vi "main_PG.vi"() -> ()   [LabVIEW 2017]
panel:
  out "P2":dbl[](array[numeric])
  out "T2":dbl[](array[numeric])
  out "V":dbl[](array[numeric])
  out "P1":dbl[](array[numeric])
  in  "Heater 2":bool
  in  "Tab Control 2":enum32{"Page 1", "Page 2"}(tab)
  in  "ON/OFF Control Loop":bool caption="Start"
  in  "Ring":u16(ring) items=["Isothermal Process", "Isochoric Process", "Boyle's Law", "Gay-Lussac Law", ""]
  in  "Exit":bool
  out "NI1":tag caption="NI device"
  out "Compressor":bool
  out "Heater":bool
  in  "Tab Control":enum32{"Page 1", "Page 2", "Page 3", "Page 4"}(tab)
  out "Air Volume (L)":dbl format="%#_3f"
  out "process":string
  in  "Save as image 6":bool
  in  "Save as Excel 6":bool
  in  "Pause Button 6":bool
  in  "Reset Chart 6":bool
  out "PV Graph":cluster{dbl[], dbl[]}(graph)
  out "Waveform Chart":cluster{"Scalar":dbl, "Scalar":dbl}(graph)
  out "Temperature":dbl(slide) caption="Temperature [C]" scale=0.0..100.0
  out "Pressure":dbl(knob) caption="Pressure [bar]" scale=-1.0..6.0
  out "Tank1":dbl(slide) scale=0.0..4.0
  in  "Save as image 5":bool
  in  "Save as Excel 5":bool
  in  "Pause Button 5":bool
  in  "Reset Chart 5":bool
  in  "Reset Chart 4":bool
  in  "Pause Button 4":bool
  in  "Save as Excel 4":bool
  in  "Save as image 4":bool
  out "Tank1 2":dbl(slide) scale=0.0..4.0
  out "Pressure 2":dbl(knob) caption="Pressure [bar]" scale=-1.0..6.0 scale format="%#_3f"
  out "Temperature 2":dbl(slide) caption="Temperature [C]" scale=0.0..100.0
  out "Waveform Chart 2":cluster{"Scalar":dbl, "Scalar":dbl}(graph)
  out "PT Graph":cluster{dbl[], dbl[]}(graph)
  in  "Reset Chart 3":bool
  in  "Pause Button 3":bool
  in  "Save as Excel 3":bool
  in  "Save as image 3":bool
  out "String":string
  out "Table":string[][](table)
  in  "BoyleNum":i64 caption="Number of samples"
  out "Total Samples":i32
  in  "BoyleNum 2":i64 caption="Number of samples"
  out "Total Samples 2":i32 caption="Total Samples"
  out "Table 2":string[][](table)
  out "String 2":string
  in  "Tab Control 3":enum32{"Page 1", "Page 2"}(tab)
  # "Expansion Processes of a Perfect Gas"
  # "Liquid Volume (L)"
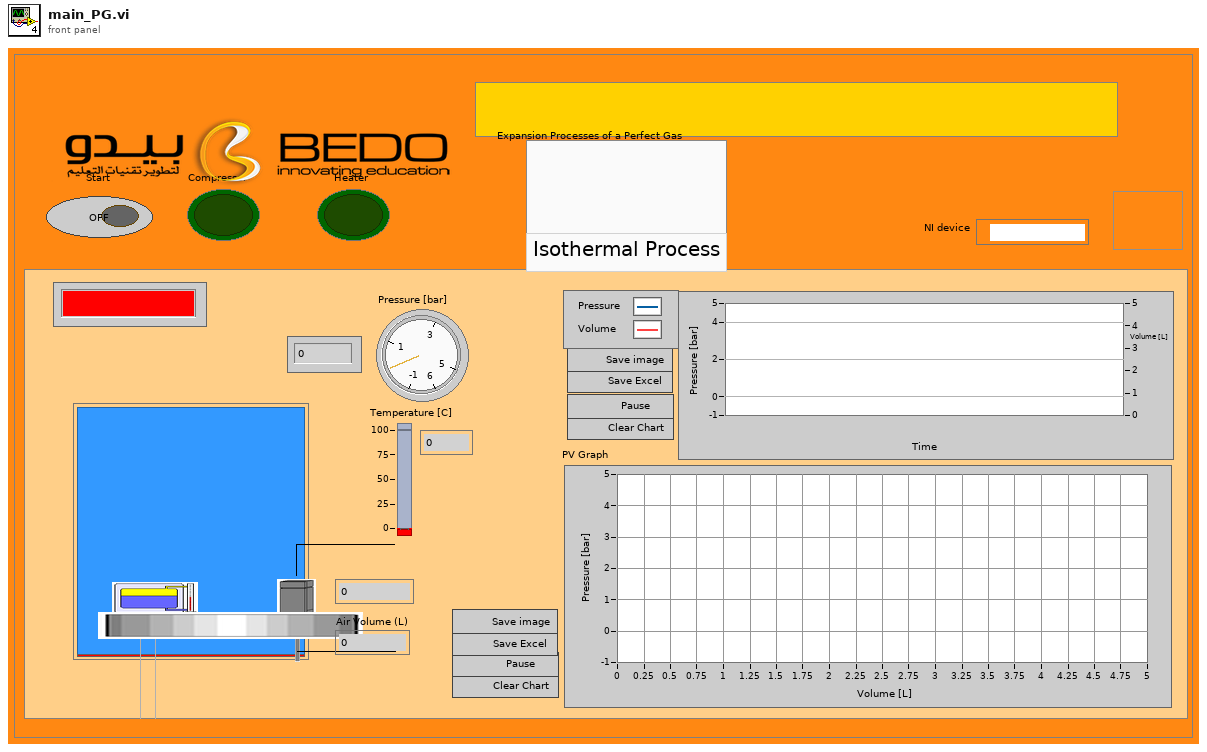
[diagram p1: front panel]
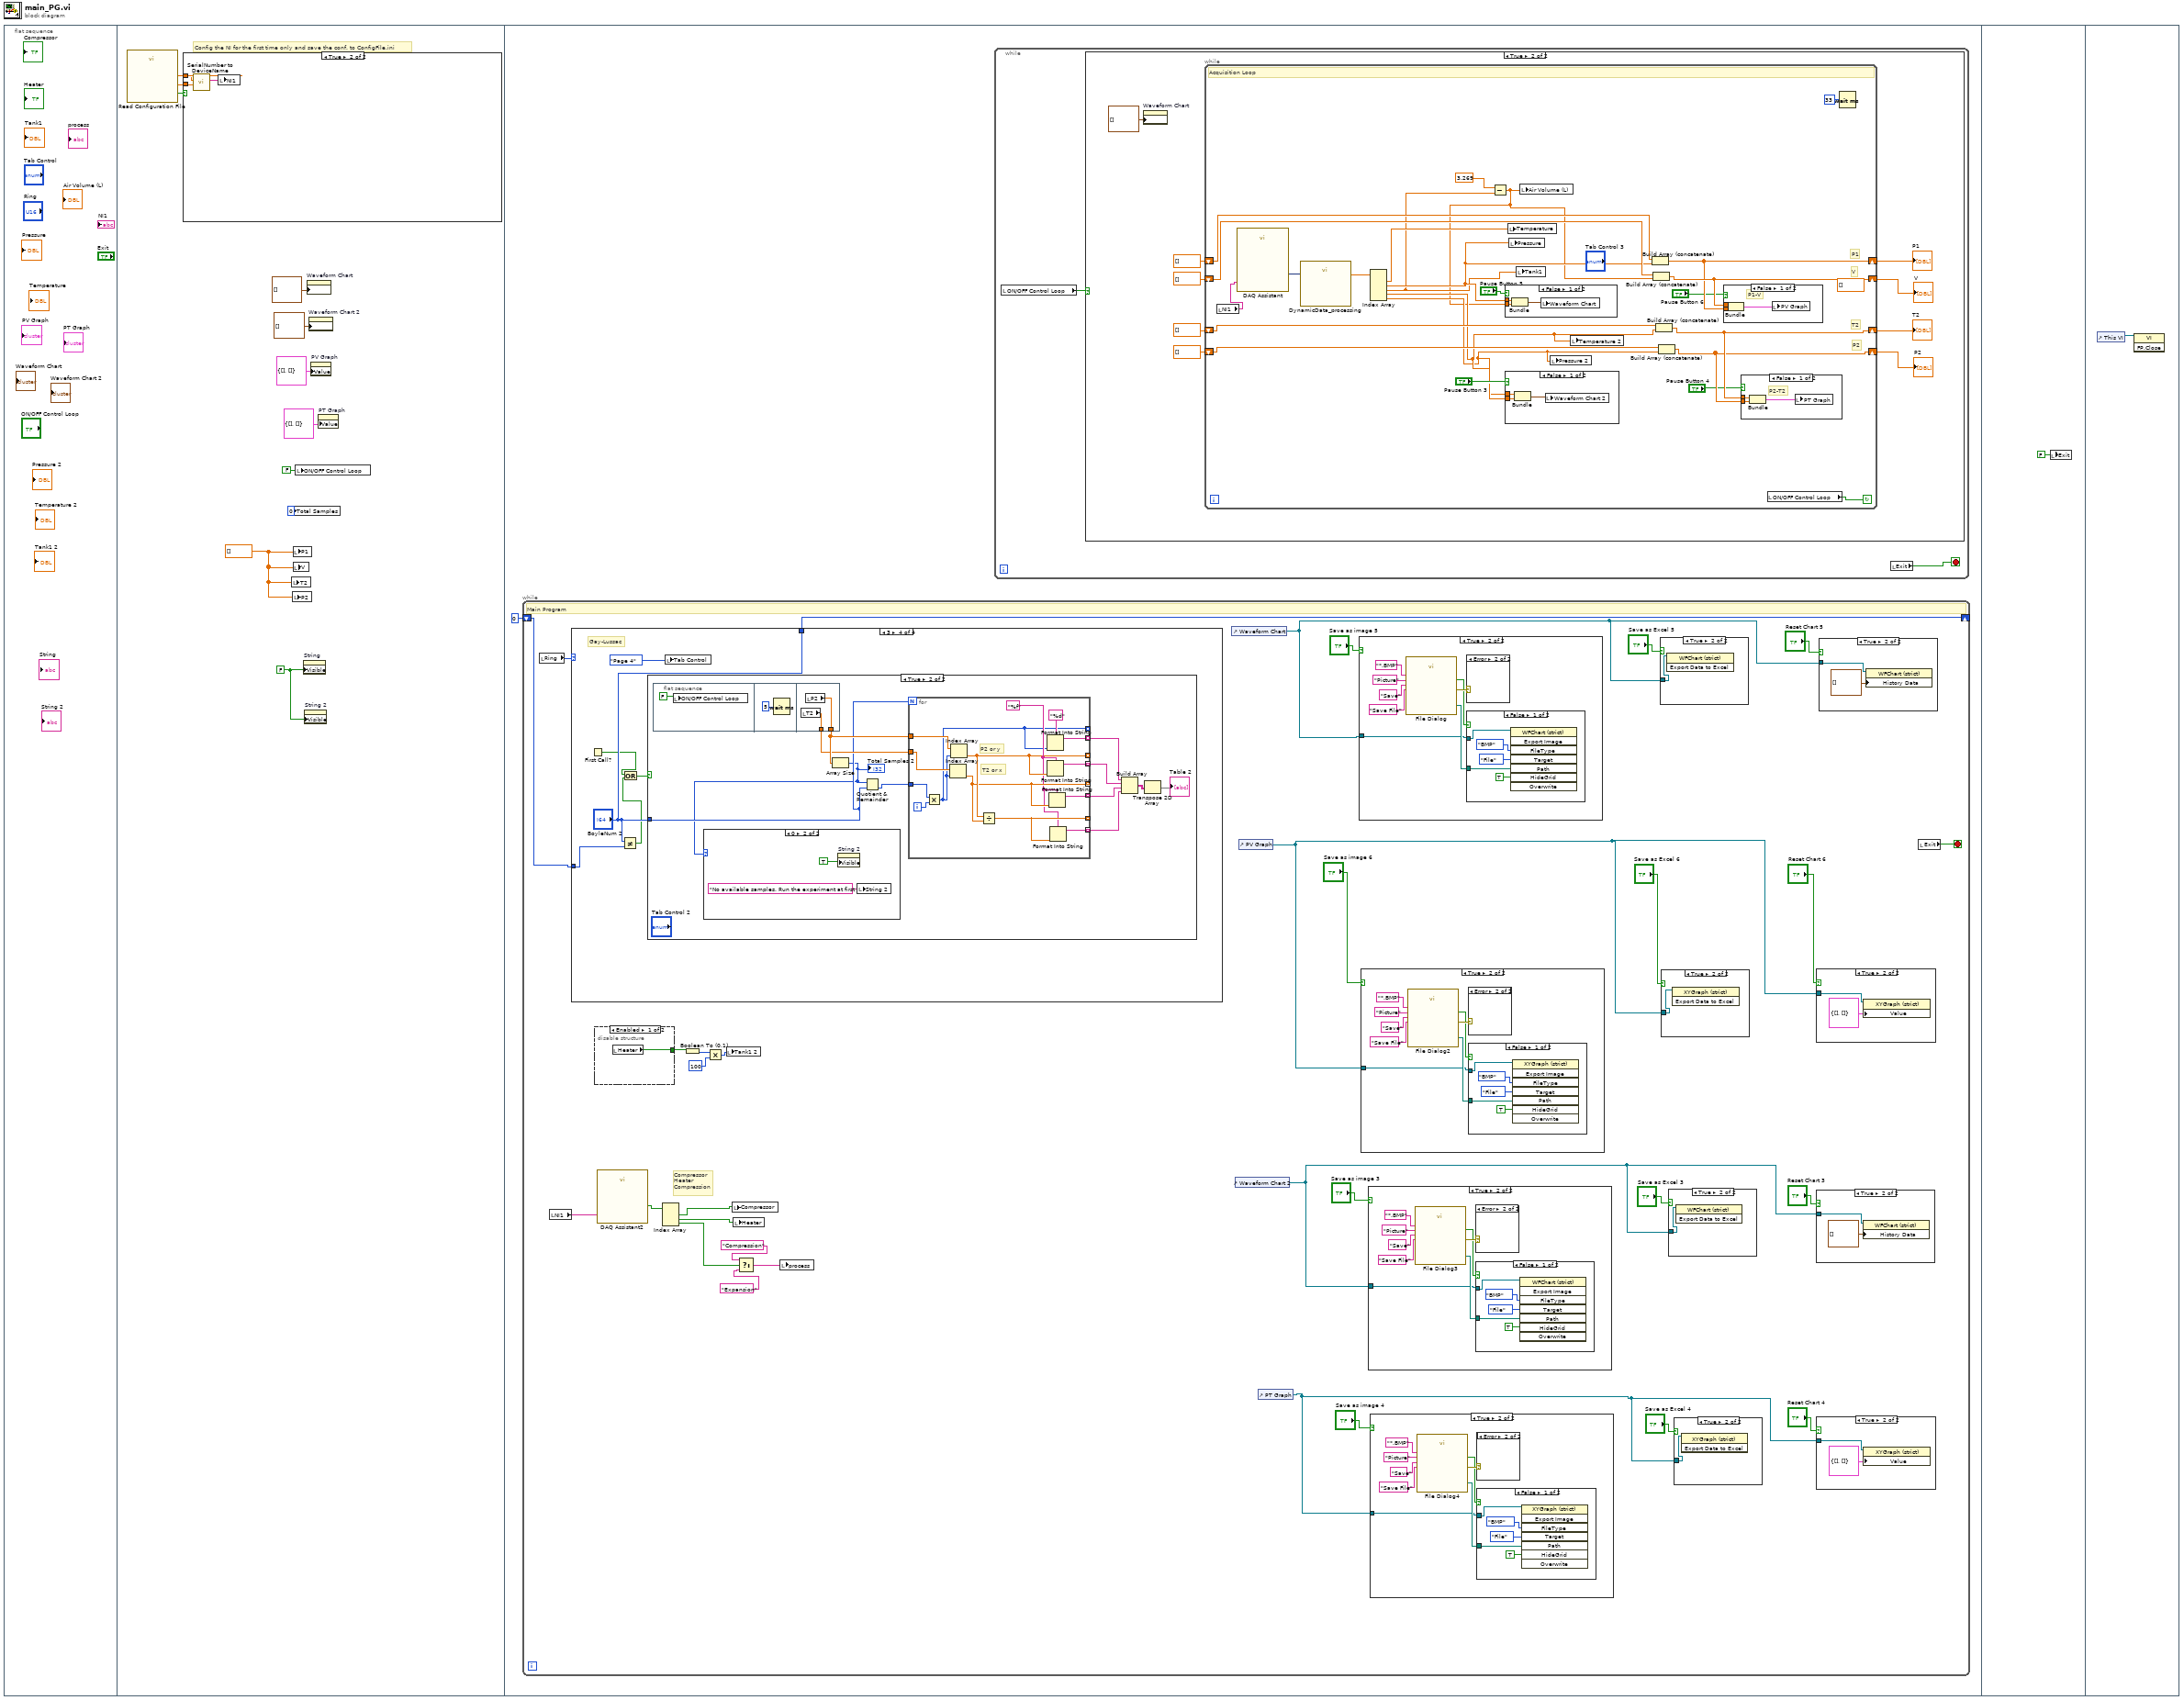
[diagram p0: block diagram]
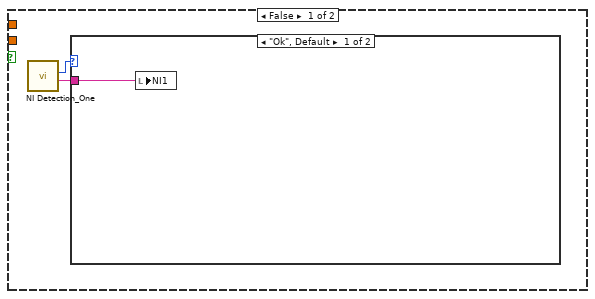
[diagram p2: hidden frame]
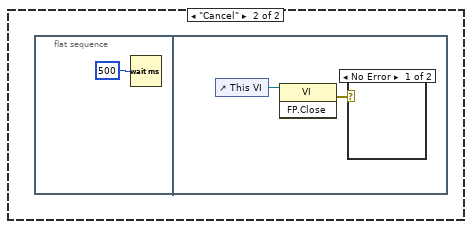
[diagram p3: hidden frame]
diagram:
  n1 = flat-sequence {
    frame #0 {
    }
    frame #1 {
      w1 = FALSE ("Visible")
      w2 = dbl[] [] ("Array")
      # "Config the NI for the first time only and save the conf. to ConfigFile.ini"
      n2 = call "Read Configuration File.vi"() -> ("Serial Numbers Found"=w9:bool, "NI1"=w10:dbl, "NI2"=w11:dbl)  [unwired: 13 in]
      n3 = case shown="True" w9 {
        tunnel: w10 -> [_ w20]
        tunnel: w11 -> [_ w19]
        frame False {
          n4 = call "NI Detection_One.vi"() -> ("NI 1"=w12:tag, "Ok/Cancel"=w13:enum16{"Ok", "Cancel"})  [unwired: 8 in, 1 out]
          n5 = case shown="\"Ok\", Default" w13 {
            tunnel: w12 -> [w14 _]
            frame "Ok", Default {
              n6 = local write "NI1"(w14) -> ()
            }
            frame "Cancel" {
              n7 = flat-sequence {
                frame #0 {
                  n8 = Wait (ms)(milliseconds to wait=u32 500) -> ()  [unwired: 1 out]
                }
                frame #1 {
                  n9 = control-ref of="This VI"() -> (w17:refnum<vi>)
                  n10 = invoke class="VI" method="FP.Close"(reference=w17) -> (error out=w16:errorcluster)  [unwired: 2 in, 2 out]
                  n11 = case shown="No Error" w16 {
                    frame No Error {
                    }
                    frame Error {
                    }
                  }
                }
              }
            }
          }
        }
        frame True {
          n12 = call "SerialNumber to DeviceName.vi"("NI2 Serial Number"=w19, "NI1 Serial Number"=w20) -> ("NI1 Device Name"=w18:tag)  [unwired: 8 in, 1 out]
          n13 = local write "NI1"(w18) -> ()
        }
      }
      n14 = local write "Total Samples"(0 ("size(s)")) -> ()
      n15 = local write "T2"(w2) -> ()
      n16 = local write "P2"(w2) -> ()
      n17 = local write "P1"(w2) -> ()
      n18 = local write "V"(w2) -> ()
      n19 = local write "ON/OFF Control Loop"(FALSE ("ON/OFF Control Loop")) -> ()
      n20 = property on="String" class="Str"("Visible"=w1) -> ()  [unwired: 2 in, 2 out]
      n21 = property on="String 2" class="Str"("Visible"=w1) -> ()  [unwired: 2 in, 2 out]
      n22 = property on="Waveform Chart" class="WFChart (strict)"("History Data"=cluster{"Scalar":dbl, "Scalar":dbl}[] []) -> ()  [unwired: 2 in, 2 out]
      n23 = property on="Waveform Chart 2" class="WFChart (strict)"("History Data"=cluster{"Scalar":dbl, "Scalar":dbl}[] []) -> ()  [unwired: 2 in, 2 out]
      n24 = property on="PV Graph" class="XYGraph (strict)"("Value"=cluster{dbl[], dbl[]} {[], []} ("PV Graph")) -> ()  [unwired: 2 in, 2 out]
      n25 = property on="PT Graph" class="XYGraph (strict)"("Value"=cluster{dbl[], dbl[]} {[], []} ("PT Graph")) -> ()  [unwired: 2 in, 2 out]
    }
    frame #2 {
      n26 = while {
        shift-right: [w31] -> _
        shift-left: i64 0 ("BoyleNum") -> [w30]
        stop <- w53 stop-if-true
        # "Compressor\nHeater\nCompression"
        # "Main Program"
        n27 = local read "Ring"() -> (w52:u16)
        n28 = local read "NI1"() -> (w29:tag)
        n29 = case shown="3" w52 {
          tunnel: [w120 w122 "BoyleNum" "BoyleNum 2"] -> w31
          tunnel: w30 -> [w120 w122 w127 w165]
          frame 0, Default {
            n30 = local write "Tab Control"(enum32{"Page 1", "Page 2"}."Page 1" ("Tab Control")) -> ()
          }
          frame 1 {
            n31 = local write "Tab Control"(enum32{"Page 1", "Page 2"}."Page 2" ("Tab Control")) -> ()
          }
          frame 2 {
            # "Boyle"
            n32 = First Call?() -> (First Call?: T/F=w124:bool)
            n33 = Not Equal?(x="BoyleNum", y=w127) -> (x != y?=w126:bool)
            n34 = Or(x=w124, y=w126) -> (x .or. y?=w125:bool)
            n35 = case shown="True" w125 {
              tunnel: "BoyleNum" -> [_ w132]
              frame False {
              }
              frame True {
                n36 = flat-sequence {
                  tunnel: [w161] -> w139
                  tunnel: [w160] -> w138
                  frame #0 {
                    n37 = local write "ON/OFF Control Loop"(FALSE ("ON/OFF Control Loop")) -> ()
                  }
                  frame #1 {
                    n38 = Wait (ms)(milliseconds to wait=u32 5) -> ()  [unwired: 1 out]
                  }
                  frame #2 {
                    n39 = local read "V"() -> (w160:dbl[])
                    n40 = local read "P1"() -> (w161:dbl[])
                  }
                }
                n41 = Array Size(array=w139) -> (size(s)=w130:i32)
                "Total Samples" <- w130
                n42 = case shown="0" w130 {
                  frame 1, Default {
                    n43 = property on="String" class="Str"("Visible"=FALSE) -> ()  [unwired: 2 in, 2 out]
                  }
                  frame 0 {
                    n44 = property on="String" class="Str"("Visible"=TRUE) -> ()  [unwired: 2 in, 2 out]
                    n45 = local write "String"("No available samples. Run the experiment at first !" ("String 2")) -> ()
                  }
                }
                n46 = Quotient & Remainder(x=w130, y=w132) -> (floor(x/y)=w140:i64)  [unwired: 1 out]
                n47 = for {
                  N: w132 -> [_]
                  tunnel: w140 -> [w157]
                  tunnel: w139 -> [w155]
                  tunnel: w138 -> [w154]
                  tunnel: [w152] -> _ mode=indexing
                  tunnel: [w150] -> _ mode=indexing
                  tunnel: [w146] -> _ mode=indexing
                  tunnel: [w149] -> _ mode=indexing
                  tunnel: [w148] -> w137 mode=indexing
                  tunnel: [w153] -> w136 mode=indexing
                  tunnel: [w151] -> w135 mode=indexing
                  tunnel: [w145] -> w131 mode=indexing
                  i -> [w146]
                  w147 = "%f" ("format string")
                  # "V or x"
                  # "P1 or y"
                  n48 = Multiply(x=w157, y=w146) -> (x*y=w156:i64)
                  n49 = Index Array(array=w154, index=w156) -> (element=w150:dbl)
                  n50 = Index Array(array=w155, index=w156) -> (element=w152:dbl)
                  n51 = Multiply(x=w152, y=w150) -> (x*y=w149:dbl)
                  n52 = Format Into String(format string=w147, w152) -> (resulting string=w148:string)  [unwired: 2 in, 1 out]
                  n53 = Format Into String(format string="%d", w146) -> (resulting string=w145:string)  [unwired: 2 in, 1 out]
                  n54 = Format Into String(format string=w147, w150) -> (resulting string=w153:string)  [unwired: 2 in, 1 out]
                  n55 = Format Into String(format string=w147, w149) -> (resulting string=w151:string)  [unwired: 2 in, 1 out]
                }
                n56 = Build Array(w131, w137, w136, w135) -> (w134:string[][])
                n57 = Transpose 2D Array(2D array=w134) -> (transposed array=→"Table":string[][])
              }
            }
            n58 = local write "Tab Control"(enum32{"Page 1", "Page 2", "Page 3", "Page 4"}."Page 3" ("Tab Control")) -> ()
          }
          frame 3 {
            # "Gay-Lussac"
            n59 = First Call?() -> (First Call?: T/F=w162:bool)
            n60 = Not Equal?(x="BoyleNum 2", y=w165) -> (x != y?=w164:bool)
            n61 = Or(x=w162, y=w164) -> (x .or. y?=w163:bool)
            n62 = case shown="True" w163 {
              tunnel: "BoyleNum 2" -> [_ w170]
              frame False {
              }
              frame True {
                n63 = flat-sequence {
                  tunnel: [w199] -> w177
                  tunnel: [w198] -> w176
                  frame #0 {
                    n64 = local write "ON/OFF Control Loop"(FALSE ("ON/OFF Control Loop")) -> ()
                  }
                  frame #1 {
                    n65 = Wait (ms)(milliseconds to wait=u32 5) -> ()  [unwired: 1 out]
                  }
                  frame #2 {
                    n66 = local read "T2"() -> (w198:dbl[])
                    n67 = local read "P2"() -> (w199:dbl[])
                  }
                }
                n68 = Array Size(array=w177) -> (size(s)=w168:i32)
                "Total Samples 2" <- w168
                n69 = case shown="0" w168 {
                  frame 1, Default {
                    n70 = property on="String 2" class="Str"("Visible"=FALSE) -> ()  [unwired: 2 in, 2 out]
                  }
                  frame 0 {
                    n71 = property on="String 2" class="Str"("Visible"=TRUE) -> ()  [unwired: 2 in, 2 out]
                    n72 = local write "String 2"("No available samples. Run the experiment at first !" ("String 2")) -> ()
                  }
                }
                n73 = Quotient & Remainder(x=w168, y=w170) -> (floor(x/y)=w178:i64)  [unwired: 1 out]
                n74 = for {
                  N: w170 -> [_]
                  tunnel: w178 -> [w195]
                  tunnel: w177 -> [w194]
                  tunnel: w176 -> [w193]
                  tunnel: [w191] -> _ mode=indexing
                  tunnel: [w189] -> _ mode=indexing
                  tunnel: [w182] -> _ mode=indexing
                  tunnel: [w188] -> _ mode=indexing
                  tunnel: [w187] -> w175 mode=indexing
                  tunnel: [w192] -> w174 mode=indexing
                  tunnel: [w190] -> w173 mode=indexing
                  tunnel: [w184] -> w169 mode=indexing
                  i -> [w185]
                  w186 = "%f" ("format string")
                  # "T2 or x"
                  # "P2 or y"
                  n75 = Multiply(x=w195, y=w185) -> (x*y=w182:i64)
                  n76 = Index Array(array=w193, index=w182) -> (element=w189:dbl)
                  n77 = Index Array(array=w194, index=w182) -> (element=w191:dbl)
                  n78 = Divide(x=w191, y=w189) -> (x/y=w188:dbl)
                  n79 = Format Into String(format string=w186, w191) -> (resulting string=w187:string)  [unwired: 2 in, 1 out]
                  n80 = Format Into String(format string="%d", w182) -> (resulting string=w184:string)  [unwired: 2 in, 1 out]
                  n81 = Format Into String(format string=w186, w189) -> (resulting string=w192:string)  [unwired: 2 in, 1 out]
                  n82 = Format Into String(format string=w186, w188) -> (resulting string=w190:string)  [unwired: 2 in, 1 out]
                }
                n83 = Build Array(w169, w175, w174, w173) -> (w172:string[][])
                n84 = Transpose 2D Array(2D array=w172) -> (transposed array=→"Table 2":string[][])
              }
            }
            n85 = local write "Tab Control"(enum32{"Page 1", "Page 2", "Page 3", "Page 4"}."Page 4" ("Tab Control")) -> ()
          }
        }
        n86 = disable-structure shown="Enabled" {
          disable-tunnel: [w118 "Heater 2"] -> w51
          frame Enabled {
            n87 = local read "Heater"() -> (w118:bool)
          }
          frame Disabled {
          }
        }
        n88 = call "DAQ Assistant2"("device name"=w29) -> ("data"=w28:bool[])  [unwired: 16 in, 2 out]
        n89 = Index Array(array=w28) -> (element #1=w27:bool, element #2=w26:bool, element #3=w25:bool)  [unwired: 3 in]
        n90 = Boolean To (0,1)(Boolean=w51) -> (0, 1=w50:i16)
        n91 = Multiply(x=w50, y=i16 100) -> (x*y=w49:i16)
        n92 = local write "Tank1 2"(w49) -> ()
        n93 = local write "Compressor"(w27) -> ()
        n94 = local write "Heater"(w26) -> ()
        n95 = Select(t="Compression", s=w25, f="Expansion") -> (s? t:f=w22:string)
        n96 = local write "process"(w22) -> ()
        n97 = control-ref of="Waveform Chart"() -> (w46:refnum<vi>)
        n98 = control-ref of="Waveform Chart 2"() -> (w36:refnum<vi>)
        n99 = control-ref of="PV Graph"() -> (w42:refnum<vi>)
        n100 = control-ref of="PT Graph"() -> (w32:refnum<vi>)
        n101 = case shown="True" "Save as image 5" {
          tunnel: w46 -> [_ w105]
          frame False {
          }
          frame True {
            n102 = call "File Dialog"("prompt"="Save File", "button label"="Save", "pattern (all files)"="*.BMP", "pattern label"="Picture") -> ("selected path"=w107:path, "cancelled"=w106:bool, "error out"=w108:errorcluster)  [unwired: 8 in, 1 out]
            n103 = case shown="Error" w108 {
              frame No Error {
              }
              frame Error {
              }
            }
            n104 = case shown="False" w106 {
              tunnel: w107 -> [w115 _]
              tunnel: w105 -> [w113 _]
              frame False {
                n105 = invoke on="Invoke Node" class="WFChart (strict)" method="Export Image"(reference=w113, "FileType"=enum32{"BMP", "EPS", "EMF", "PICT"}."BMP" ("File Type"), "Target"=enum32{"File", "Clipboard"}."File", "Path"=w115, "HideGrid"=TRUE ("Hide Grid")) -> ()  [unwired: 3 in, 8 out]
              }
              frame True {
              }
            }
          }
        }
        n106 = case shown="True" "Save as image 6" {
          tunnel: w42 -> [_ w89]
          frame False {
          }
          frame True {
            n107 = call "File Dialog2"("prompt"="Save File", "button label"="Save", "pattern (all files)"="*.BMP", "pattern label"="Picture") -> ("selected path"=w91:path, "cancelled"=w90:bool, "error out"=w92:errorcluster)  [unwired: 8 in, 1 out]
            n108 = case shown="Error" w92 {
              frame No Error {
              }
              frame Error {
              }
            }
            n109 = case shown="False" w90 {
              tunnel: w91 -> [w99 _]
              tunnel: w89 -> [w97 _]
              frame False {
                n110 = invoke on="Invoke Node" class="XYGraph (strict)" method="Export Image"(reference=w97, "FileType"=enum32{"BMP", "EPS", "EMF", "PICT"}."BMP" ("File Type"), "Target"=enum32{"File", "Clipboard"}."File", "Path"=w99, "HideGrid"=TRUE ("Hide Grid")) -> ()  [unwired: 3 in, 8 out]
              }
              frame True {
              }
            }
          }
        }
        n111 = case shown="True" "Save as image 3" {
          tunnel: w36 -> [_ w73]
          frame False {
          }
          frame True {
            n112 = call "File Dialog3"("prompt"="Save File", "button label"="Save", "pattern (all files)"="*.BMP", "pattern label"="Picture") -> ("selected path"=w75:path, "cancelled"=w74:bool, "error out"=w76:errorcluster)  [unwired: 8 in, 1 out]
            n113 = case shown="Error" w76 {
              frame No Error {
              }
              frame Error {
              }
            }
            n114 = case shown="False" w74 {
              tunnel: w75 -> [w83 _]
              tunnel: w73 -> [w81 _]
              frame False {
                n115 = invoke on="Invoke Node" class="WFChart (strict)" method="Export Image"(reference=w81, "FileType"=enum32{"BMP", "EPS", "EMF", "PICT"}."BMP" ("File Type"), "Target"=enum32{"File", "Clipboard"}."File", "Path"=w83, "HideGrid"=TRUE ("Hide Grid")) -> ()  [unwired: 3 in, 8 out]
              }
              frame True {
              }
            }
          }
        }
        n116 = case shown="True" "Save as image 4" {
          tunnel: w32 -> [_ w57]
          frame False {
          }
          frame True {
            n117 = call "File Dialog4"("prompt"="Save File", "button label"="Save", "pattern (all files)"="*.BMP", "pattern label"="Picture") -> ("selected path"=w59:path, "cancelled"=w58:bool, "error out"=w60:errorcluster)  [unwired: 8 in, 1 out]
            n118 = case shown="Error" w60 {
              frame No Error {
              }
              frame Error {
              }
            }
            n119 = case shown="False" w58 {
              tunnel: w59 -> [w67 _]
              tunnel: w57 -> [w65 _]
              frame False {
                n120 = invoke on="Invoke Node" class="XYGraph (strict)" method="Export Image"(reference=w65, "FileType"=enum32{"BMP", "EPS", "EMF", "PICT"}."BMP" ("File Type"), "Target"=enum32{"File", "Clipboard"}."File", "Path"=w67, "HideGrid"=TRUE ("Hide Grid")) -> ()  [unwired: 3 in, 8 out]
              }
              frame True {
              }
            }
          }
        }
        n121 = case shown="True" "Save as Excel 5" {
          tunnel: w46 -> [_ w104]
          frame False {
          }
          frame True {
            n122 = invoke on="Invoke Node" class="WFChart (strict)" method="Export Data to Excel"(reference=w104) -> ()  [unwired: 2 in, 3 out]
          }
        }
        n123 = case shown="True" "Save as Excel 6" {
          tunnel: w42 -> [_ w88]
          frame False {
          }
          frame True {
            n124 = invoke on="Invoke Node" class="XYGraph (strict)" method="Export Data to Excel"(reference=w88) -> ()  [unwired: 2 in, 3 out]
          }
        }
        n125 = case shown="True" "Save as Excel 3" {
          tunnel: w36 -> [_ w72]
          frame False {
          }
          frame True {
            n126 = invoke on="Invoke Node" class="WFChart (strict)" method="Export Data to Excel"(reference=w72) -> ()  [unwired: 2 in, 3 out]
          }
        }
        n127 = case shown="True" "Save as Excel 4" {
          tunnel: w32 -> [_ w56]
          frame False {
          }
          frame True {
            n128 = invoke on="Invoke Node" class="XYGraph (strict)" method="Export Data to Excel"(reference=w56) -> ()  [unwired: 2 in, 3 out]
          }
        }
        n129 = case shown="True" "Reset Chart 3" {
          tunnel: w36 -> [_ w71]
          frame False {
          }
          frame True {
            n130 = property on="Property Node" class="WFChart (strict)"(reference=w71, "History Data"=cluster{"Scalar":dbl, "Scalar":dbl}[] []) -> ()  [unwired: 1 in, 2 out]
          }
        }
        n131 = case shown="True" "Reset Chart 6" {
          tunnel: w42 -> [_ w87]
          frame False {
          }
          frame True {
            n132 = property on="Property Node" class="XYGraph (strict)"(reference=w87, "Value"=cluster{dbl[], dbl[]} {[], []}) -> ()  [unwired: 1 in, 2 out]
          }
        }
        n133 = case shown="True" "Reset Chart 4" {
          tunnel: w32 -> [_ w55]
          frame False {
          }
          frame True {
            n134 = property on="Property Node" class="XYGraph (strict)"(reference=w55, "Value"=cluster{dbl[], dbl[]} {[], []}) -> ()  [unwired: 1 in, 2 out]
          }
        }
        n135 = case shown="True" "Reset Chart 5" {
          tunnel: w46 -> [_ w103]
          frame False {
          }
          frame True {
            n136 = property on="Property Node" class="WFChart (strict)"(reference=w103, "History Data"=cluster{"Scalar":dbl, "Scalar":dbl}[] []) -> ()  [unwired: 1 in, 2 out]
          }
        }
        n137 = local read "Exit"() -> (w53:bool)
      }
      n138 = while {
        stop <- w200 stop-if-true
        n139 = local read "ON/OFF Control Loop"() -> (w201:bool)
        n140 = case shown="True" w201 {
          frame False {
          }
          frame True {
            n141 = property on="Waveform Chart" class="WFChart (strict)"("History Data"=cluster{"Scalar":dbl, "Scalar":dbl}[] []) -> ()  [unwired: 2 in, 2 out]
            n142 = while {
              shift-right: [w222] -> w205
              shift-left: dbl[] [] -> [w231]
              shift-right: [w223] -> w204
              shift-left: dbl[] [] -> [w230]
              shift-right: [w221] -> w203
              shift-left: dbl[] [] -> [w226]
              shift-right: [w220] -> w202
              shift-left: dbl[] [] -> [w225]
              stop <- w229 continue-if-true
              (unwired) dbl[] []
              # "P2"
              # "T2"
              # "V"
              # "P1"
              # "Acquisition Loop"
              n143 = local read "NI1"() -> (w228:tag)
              n144 = call "DAQ Assistant"("device name"=w228) -> ("data"=w233:dynamicdata)  [unwired: 16 in, 2 out]
              n145 = call "DynamicData_processing.vi"("data"=w233) -> ("DATA"=w234:dbl[])
              n146 = Index Array(array=w234) -> (element #1=w227:dbl, element #2=w224:dbl, element #3=w212:dbl, element #4=w215:dbl, element #5=w214:dbl)  [unwired: 5 in]
              n147 = Subtract(x=3.269 ("y"), y=w212) -> (x-y=w211:dbl)
              n148 = case shown="False" "Pause Button 5" {
                tunnel: w224 -> [w245 _]
                tunnel: w211 -> [w244 _]
                frame False {
                  n149 = Bundle("Scalar"=w245, w244) -> (w246:cluster{"Scalar":dbl, dbl})  [unwired: 1 in]
                  n150 = local write "Waveform Chart"(w246) -> ()
                }
                frame True {
                }
              }
              n151 = case shown="False" "Pause Button 3" {
                tunnel: w214 -> [w239 _]
                tunnel: w215 -> [w238 _]
                frame False {
                  n152 = Bundle("Scalar"=w239, "Scalar"=w238) -> (w240:cluster{"Scalar":dbl, "Scalar":dbl})  [unwired: 1 in]
                  n153 = local write "Waveform Chart 2"(w240) -> ()
                }
                frame True {
                }
              }
              n154 = local write "Temperature"(w227) -> ()
              n155 = local write "Pressure"(w224) -> ()
              n156 = local write "Tank1"(w212) -> ()
              n157 = local write "Air Volume (L)"(w211) -> ()
              n158 = local write "Pressure 2"(w214) -> ()
              n159 = local write "Temperature 2"(w215) -> ()
              n160 = Build Array (concatenate)(w231, w224) -> (w222:dbl[])
              n161 = Build Array (concatenate)(w230, w211) -> (w223:dbl[])
              n162 = Build Array (concatenate)(w226, w215) -> (w221:dbl[])
              n163 = Build Array (concatenate)(w225, w214) -> (w220:dbl[])
              n164 = case shown="False" "Pause Button 6" {
                tunnel: w223 -> [w242 _]
                tunnel: w222 -> [w241 _]
                frame False {
                  # "P1-V"
                  n165 = Bundle(w242, w241) -> (w243:cluster{dbl[], dbl[]})  [unwired: 1 in]
                  n166 = local write "PV Graph"(w243) -> ()
                }
                frame True {
                }
              }
              n167 = case shown="False" "Pause Button 4" {
                tunnel: w221 -> [w237 _]
                tunnel: w220 -> [w236 _]
                frame False {
                  # "P2-T2"
                  n168 = Bundle(w237, w236) -> (w235:cluster{dbl[], dbl[]})  [unwired: 1 in]
                  n169 = local write "PT Graph"(w235) -> ()
                }
                frame True {
                }
              }
              n170 = local read "ON/OFF Control Loop"() -> (w229:bool)
              n171 = Wait (ms)(milliseconds to wait=u32 33) -> ()  [unwired: 1 out]
            }
            "P1" <- w205
            "V" <- w204
            "T2" <- w203
            "P2" <- w202
          }
        }
        n172 = local read "Exit"() -> (w200:bool)
      }
    }
    frame #3 {
      n173 = local write "Exit"(FALSE ("Exit")) -> ()
    }
    frame #4 {
      n174 = control-ref of="This VI"() -> (w248:refnum<vi>)
      n175 = invoke class="VI" method="FP.Close"(reference=w248) -> ()  [unwired: 2 in, 3 out]
    }
  }
